vi "terminate.vi"(8 "error in (no error)":errorcluster, 11 "DL090202ScanHead in":refnum<class "ScanHeadDL090202.lvclass">) -> (0 "error out":errorcluster, 3 "DL090202ScanHead out":refnum<class "ScanHeadDL090202.lvclass">)   [LabVIEW 2010, in "ScanHeadDL090202.lvclass"]
uses:
  ScanHeadDL090202.lvclass
  DigitalOut/GenericDigitalOut/GenericDigitalOut/GenericDigitalOut.lvclass
  Clock/GenericClock/GenericClock/GenericClock.lvclass
  GenericScanHead/GenericScanHead/GenericScanHead.lvclass
  common/classes/ErrorController/ErrorController/class_data.vi
  common/classes/ErrorController/ErrorController/ErrorController.lvclass
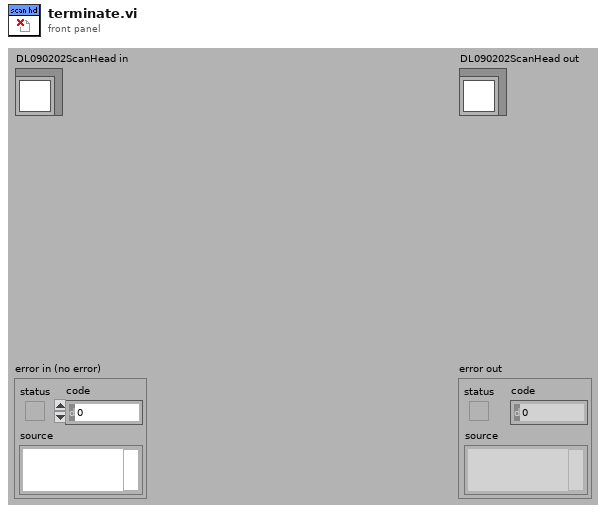
[diagram p1: front panel]
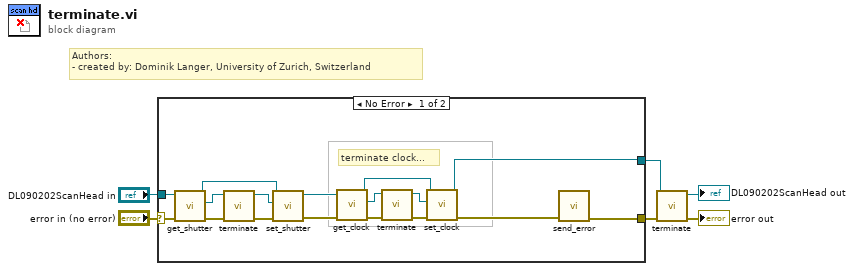
[diagram p0: block diagram]
diagram:
  # "Authors: \n- created by: Dominik Langer, University of Zurich, Switzerland"
  n1 = case shown="No Error" "error in (no error)" {
    selector: "error in (no error)" -> [w16 w25]
    tunnel: [w18 w25] -> w4
    tunnel: [w7 w24] -> w3
    tunnel: "DL090202ScanHead in" -> [w17 w24]
    frame No Error {
      # "terminate clock..."
      n2 = call-dynamic "get_shutter.vi"("error in (no error)"=w16, "DL090202ScanHead.lvclass in"=w17) -> ("error out"=w21:errorcluster, "GenericDigitalOut.lvclass"=w20:refnum<class "GenericDigitalOut.lvclass">, "DL090202ScanHead.lvclass out"=w22:refnum<class "ScanHeadDL090202.lvclass">)  [unwired: 7 out]
      n3 = call-dynamic "terminate.vi"("error in (no error)"=w21, "GenericPlugin in"=w20) -> ("error out"=w23:errorcluster, "GenericPlugin out"=w19:refnum<class "GenericDigitalOut.lvclass">)  [unwired: 8 out]
      n4 = call-dynamic "set_shutter.vi"("error in (no error)"=w23, "GenericDigitalOut.lvclass"=w19, "DL090202ScanHead.lvclass in"=w22) -> ("error out"=w10:errorcluster, "DL090202ScanHead.lvclass out"=w8:refnum<class "ScanHeadDL090202.lvclass">)  [unwired: 7 out]
      n5 = call-dynamic "get_clock.vi"("error in (no error)"=w10, "DL090202ScanHead.lvclass in"=w8) -> ("error out"=w14:errorcluster, "GenericClock.lvclass"=w13:refnum<class "GenericClock.lvclass">, "DL090202ScanHead.lvclass out"=w11:refnum<class "ScanHeadDL090202.lvclass">)  [unwired: 7 out]
      n6 = call-dynamic "terminate.vi"("error in (no error)"=w14, "GenericPlugin in"=w13) -> ("error out"=w15:errorcluster, "GenericPlugin out"=w12:refnum<class "GenericClock.lvclass">)  [unwired: 8 out]
      n7 = call-dynamic "set_clock.vi"("error in (no error)"=w15, "GenericClock.lvclass"=w12, "DL090202ScanHead.lvclass in"=w11) -> ("error out"=w9:errorcluster, "DL090202ScanHead.lvclass out"=w7:refnum<class "ScanHeadDL090202.lvclass">)  [unwired: 7 out]
      n8 = call "send_error.vi"("error in (no error)"=w9) -> ("error out"=w18:errorcluster)  [unwired: 10 in]
    }
    frame Error {
    }
  }
  n9 = call-parent "terminate.vi"("error in (no error)"=w4, "GenericPlugin in"=w3) -> ("error out"=→"error out":errorcluster, "GenericPlugin out"=→"DL090202ScanHead out":refnum<class "ScanHeadDL090202.lvclass">)  [unwired: 8 in]
